vi "OpenDrive.vi"(8 "error in":errorcluster) -> (0 "error out":errorcluster, 2 "Calibrated":bool, 3 "RobotDriveDevRef":T1={"DevStatus"={"status"=FALSE, "code"=0, "source"=""}, "Motors[]"=[], "Square Inputs"=FALSE, "Max Output"=1.0})   [LabVIEW 2020]
uses:
  <vilib>/Rock Robotics/WPI/RobotDrive/WPI_RobotDriveDevRef.ctl
  <vilib>/Rock Robotics/WPI/MotorControl/WPI_MotorControlDeviceRef.ctl
  <vilib>/Rock Robotics/WPI/MotorControl/WPI_MotorControlType.ctl
  <vilib>/Rock Robotics/SystemInterfaces/DIO/FPGA_DIOPWMChannel.ctl
  <vilib>/Rock Robotics/WPI/PWM/WPI_PWMDeadband.ctl
  <vilib>/Rock Robotics/SystemInterfaces/DIO/FPGA_DIOChannel.ctl
  <vilib>/Rock Robotics/WPI/ThirdParty/Phoenix-LabVIEW/Motor Controller/Controls/CTRE_Phoenix_MotorControl_NeutralMode.ctl
  <vilib>/Rock Robotics/WPI/Encoder/WPI_EncoderType.ctl
  <vilib>/Rock Robotics/WPI/SafetyOutput/WPI_SafetyOutputConfigMenu.ctl
  <vilib>/Rock Robotics/WPI/Counter/WPI_CounterDigitalInputToDigitalSource.vi
  <vilib>/Rock Robotics/WPI/Counter/WPI_CounterOpen Semi Period Mode.vi
  <vilib>/Rock Robotics/WPI/RobotDrive/WPI_RobotDriveOpen2MotorWithExistingMotors.vi
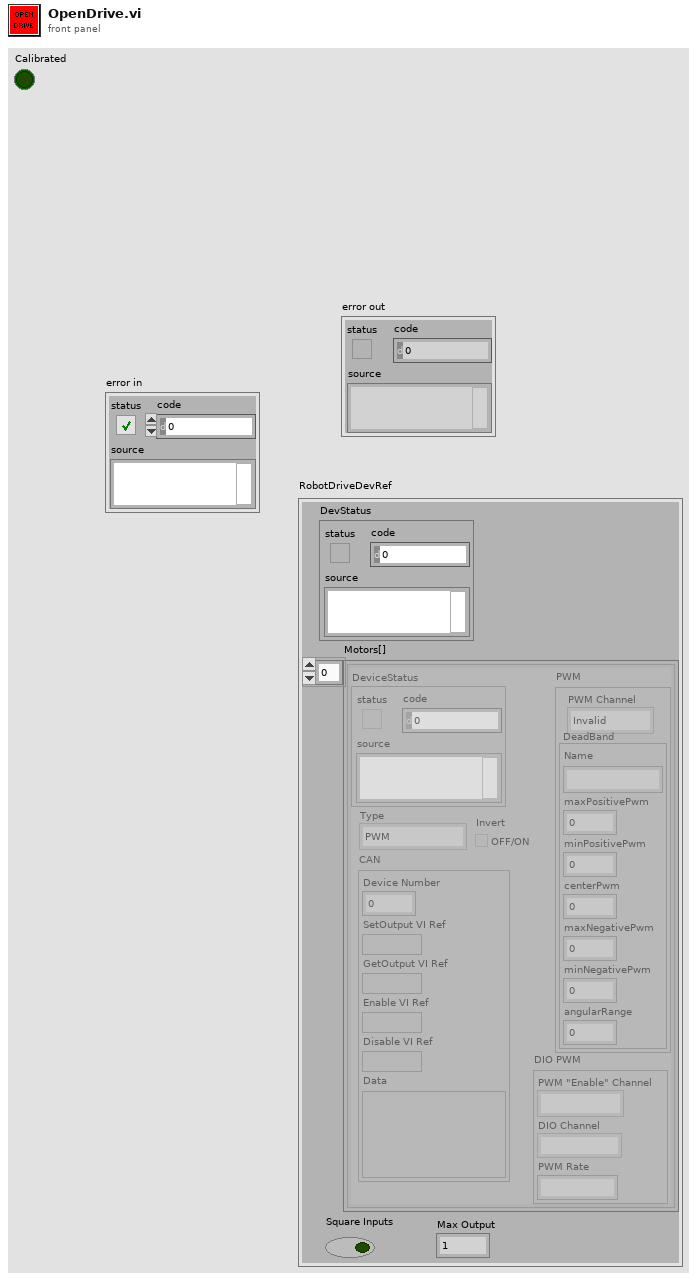
[diagram p1: front panel]
types:
  T1 = typedef "WPI_RobotDriveDevRef.ctl" = cluster{"DevStatus":errorcluster, "Motors[]":T2[], "Square Inputs":bool, "Max Output":dbl}
  T2 = typedef "WPI_MotorControlDeviceRef.ctl" = cluster{"DeviceStatus":errorcluster, "Type":T3, "PWM":cluster{"PWM Channel":T4, "DeadBand":T5}, "CAN":cluster{"Device Number":u8, "SetOutput VI Ref":variant, "GetOutput VI Ref":variant, "Enable VI Ref":variant, "Disable VI Ref":variant, "Data":variant}, "Invert":bool, "DIO PWM":cluster{"PWM \"Enable\" Channel":T4, "DIOChannel":T6, "PWM Rate":dbl}}
  T3 = typedef "WPI_MotorControlType.ctl" = enum16{"PWM", "CAN", "DIO PWM"}
  T4 = typedef "FPGA_DIOPWMChannel.ctl" = enum8{"PWM 0", "PWM 1", "PWM 2", "PWM 3", "PWM 4", "PWM 5", "PWM 6", "PWM 7", "PWM 8", "PWM 9", "PWM MXP 0", "PWM MXP 1", "PWM MXP 2", "PWM MXP 3", "PWM MXP 4", "PWM MXP 5", "PWM MXP 6", "PWM MXP 7", "PWM MXP 8", "PWM MXP 9", "Invalid"}
  T5 = typedef "WPI_PWMDeadband.ctl" = cluster{"Name":string, "maxPositivePwm":i32, "minPositivePwm":i32, "centerPwm":i32, "maxNegativePwm":i32, "minNegativePwm":i32, "angularRange":u16}
  T6 = typedef "FPGA_DIOChannel.ctl" = enum8{"DIO 0", "DIO 1", "DIO 2", "DIO 3", "DIO 4", "DIO 5", "DIO 6", "DIO 7", "DIO 8", "DIO 9", "DIO MXP 0", "DIO MXP 1", "DIO MXP 2", "DIO MXP 3", "DIO MXP 4", "DIO MXP 5", "DIO MXP 6", "DIO MXP 7", "DIO MXP 8", "DIO MXP 9", "DIO MXP 10", "DIO MXP 11", "DIO MXP 12", "DIO MXP 13", "DIO MXP 14", "DIO MXP 15", "SPI Port CS1", "SPI Port CS2", "SPI Port CS3", "SPI Port MISO", "SPI Port MOSI", "Invalid"}
  T7 = typedef "CTRE_Phoenix_MotorControl_NeutralMode.ctl" = enum8{"EEPROMSetting", "Override to Coast", "Override to Brake"}
  T8 = typedef "WPI_EncoderType.ctl" = enum16{"1x", "2x", "4x"}
  T9 = typedef "WPI_SafetyOutputConfigMenu.ctl" = enum16{"Enable", "Disable"}
  T10 = typedef "WPI_DigitalInputDevRef.ctl" = cluster{"DevStatus":errorcluster, "DIO Channel":T6}
  T11 = typedef "FPGA_CounterEncoderSourceConvertionLVSourceType.ctl" = cluster{"DevStatus":errorcluster, "AnalogTriggerMode?":bool, "DigitalMode":cluster{"DIO Channel":T12}, "AnalogTriggerMode":cluster{"AnalogTriggerIndex":T13, "OutputType":T14}}
  T12 = typedef "FPGA_DIODigitalSourceChannel.ctl" = enum8{"DIO 0", "DIO 1", "DIO 2", "DIO 3", "DIO 4", "DIO 5", "DIO 6", "DIO 7", "DIO 8", "DIO 9", "DIO MXP 0", "DIO MXP 1", "DIO MXP 2", "DIO MXP 3", "DIO MXP 4", "DIO MXP 5", "DIO MXP 6", "DIO MXP 7", "DIO MXP 8", "DIO MXP 9", "DIO MXP 10", "DIO MXP 11", "DIO MXP 12", "DIO MXP 13", "DIO MXP 14", "DIO MXP 15", "SPI Port CS1", "SPI Port CS2", "SPI Port CS3", "SPI Port MISO", "SPI Port MOSI", "Disabled"}
  T13 = typedef "FPGA_AnalogTriggerIndex.ctl" = enum8{"Trig 0", "Trig 1", "Trig 2", "Trig 3", "Trig 4", "Trig 5", "Trig 6", "Trig 7", "Invalid"}
  T14 = typedef "FPGA_AnalogTriggerOutType.ctl" = enum16{"InWindow", "TriggerState", "Rising", "Falling"}
  T15 = typedef "WPI_CounterDevRef.ctl" = cluster{"DevStatus":errorcluster, "CntIndex":T16}
  T16 = typedef "FPGA_CounterCtrSystemIndex.ctl" = enum8{"Ctr 0", "Ctr 1", "Ctr 2", "Ctr 3", "Ctr 4", "Ctr 5", "Ctr 6", "Ctr 7", "Invalid"}
  T17 = typedef "WPI_EncoderDevRef.ctl" = cluster{"DevStatus":errorcluster, "EncoderIndex":T18, "CounterIndex":T16, "DistancePerCount":dbl, "Decoding Type":T8}
  T18 = typedef "FPGA_EncoderIdx.ctl" = enum8{"Enc 0", "Enc 1", "Enc 2", "Enc 3", "Enc 4", "Enc 5", "Enc 6", "Enc 7", "Invalid"}
  T19 = typedef "ADIS16470 Device Reference.ctl" = cluster{"DevStatus":errorcluster, "Hardware Config":T20, "Calibration Complete":refnum<notifier>, "Status Reference":refnum<data-value>, "Data Reference":refnum<data-value>, "Sychronous Process VI":T23, "Cmd FIFO":refnum<k33>, "Source":T11, "Data FIFO":refnum<k33>, "Calibration Time (ms)":u32, "Data Reference":refnum<data-value>}
  T20 = typedef "ADIS16470 Hardware Configuration.ctl" = cluster{"SPI Clock Rate (Hz)":dbl, "IMU SPI Mode (3)":T21, "IMU Reset Pin":T6, "IMU SPI Bus":T22, "IMU Data Ready Pin":T6, "Stall Config":cluster{"Pow2BytesPerRead":u8, "StallTicks":u16, "CsToSclkTicks":u8}}
  T21 = typedef "WPI_SPIMode.ctl" = enum16{"Mode 0 (Clk Idle Low,Sample on Leading)", "Mode 1 (Clk Idle Low,Sample on Trailing)", "Mode 2 (Clk Idle High,Sample on Leading)", "Mode 3 (Clk Idle High,Sample on Trailing)"}
  T22 = typedef "spi_bus.ctl" = enum16{"SPI On-Board, CS0", "SPI On-Board, CS1", "SPI On-Board, CS2", "SPI On-Board, CS3", "SPI MXP", "Invalid"}
  T23 = typedef "ADIS16470 Process.ctl" = refnum<vi>
  T24 = typedef "ADIS16470 Status.ctl" = cluster{"Calibrated?":bool, "IMU Detected?":bool}
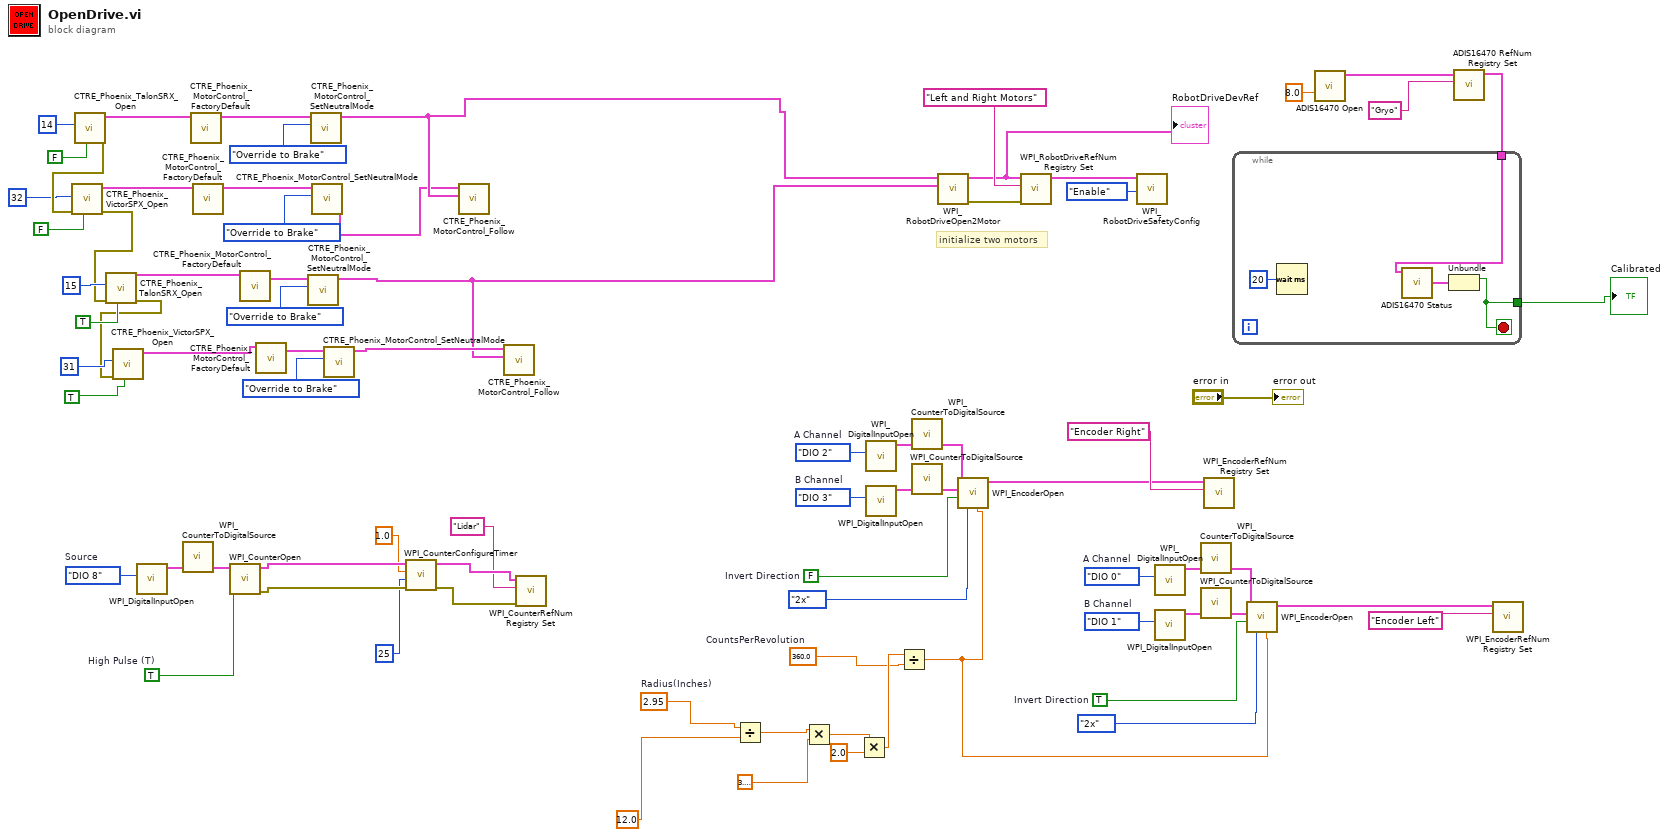
[diagram p0: block diagram]
diagram:
  w29 = TRUE  # High Pulse (T)
  w38 = FPGA_DIOChannel."DIO 8"  # Source
  w43 = 2.95  # Radius(Inches)
  w53 = TRUE  # Invert Direction
  w57 = FPGA_DIOChannel."DIO 1"  # B Channel
  w56 = FPGA_DIOChannel."DIO 0"  # A Channel
  w45 = 360.0  # CountsPerRevolution
  w63 = FALSE  # Invert Direction
  w67 = FPGA_DIOChannel."DIO 3"  # B Channel
  w66 = FPGA_DIOChannel."DIO 2"  # A Channel
  # "initialize two motors"
  n1 = call <vilib>:"CTRE_Phoenix_TalonSRX_Open.vi"("Invert"=FALSE, "Device Number"=u8 14) -> ("error out"=w15:errorcluster, "PhoenixMotorControlDevRef"=w20:T2)  [unwired: 8 in]
  n2 = call <vilib>:"CTRE_Phoenix_VictorSPX_Open.vi"("Invert"=FALSE, "error in"=w15, "Device Number"=u8 32) -> ("error out"=w14:errorcluster, "PhoenixMotorControlDevRef"=w11:T2)  [unwired: 7 in]
  n3 = call <vilib>:"CTRE_Phoenix_TalonSRX_Open.vi"("Invert"=TRUE, "error in"=w14, "Device Number"=u8 15) -> ("error out"=w7:errorcluster, "PhoenixMotorControlDevRef"=w26:T2)  [unwired: 7 in]
  n4 = call <vilib>:"CTRE_Phoenix_VictorSPX_Open.vi"("Invert"=TRUE, "error in"=w7, "Device Number"=u8 31) -> ("PhoenixMotorControlDevRef"=w10:T2)  [unwired: 7 in, 1 out]
  n5 = call <vilib>:"WPI_DigitalInputOpen.vi"("DIO Channel"=w38) -> ("DigitalInputDevRef"=w37:T10)  [unwired: 1 in, 9 out]
  n6 = call-poly <vilib>:"WPI_CounterToDigitalSource.vi"("DigitalInputDevRef"=w37) -> ("Digital Source"=w39:T11)  [unwired: 6 out]
  n7 = call <vilib>:"CTRE_Phoenix_MotorControl_FactoryDefault.vi"("PhoenixMotorControlDevRef"=w20) -> ("PhoenixMotorControlDevRef"=w21:T2)  [unwired: 9 in, 1 out]
  n8 = call <vilib>:"CTRE_Phoenix_MotorControl_FactoryDefault.vi"("PhoenixMotorControlDevRef"=w11) -> ("PhoenixMotorControlDevRef"=w17:T2)  [unwired: 9 in, 1 out]
  n9 = call-poly <vilib>:"WPI_CounterOpen.vi"("High Pulse (T)"=w29, "Source"=w39) -> ("error out"=w33:errorcluster, "CounterDevRef"=w36:T15)  [unwired: 3 in, 5 out]
  n10 = call <vilib>:"CTRE_Phoenix_MotorControl_FactoryDefault.vi"("PhoenixMotorControlDevRef"=w26) -> ("PhoenixMotorControlDevRef"=w27:T2)  [unwired: 9 in, 1 out]
  n11 = call <vilib>:"CTRE_Phoenix_MotorControl_FactoryDefault.vi"("PhoenixMotorControlDevRef"=w10) -> ("PhoenixMotorControlDevRef"=w24:T2)  [unwired: 9 in, 1 out]
  n12 = call <vilib>:"CTRE_Phoenix_MotorControl_SetNeutralMode.vi"("Motor Control Neutral Mode"=CTRE_Phoenix_MotorControl_NeutralMode."Override to Brake", "PhoenixMotorControlDevRef"=w27) -> ("PhoenixMotorControlDevRef"=w6:T2)  [unwired: 8 in, 1 out]
  n13 = call <vilib>:"CTRE_Phoenix_MotorControl_SetNeutralMode.vi"("Motor Control Neutral Mode"=CTRE_Phoenix_MotorControl_NeutralMode."Override to Brake", "PhoenixMotorControlDevRef"=w21) -> ("PhoenixMotorControlDevRef"=w19:T2)  [unwired: 8 in, 1 out]
  n14 = call <vilib>:"CTRE_Phoenix_MotorControl_SetNeutralMode.vi"("Motor Control Neutral Mode"=CTRE_Phoenix_MotorControl_NeutralMode."Override to Brake", "PhoenixMotorControlDevRef"=w17) -> ("PhoenixMotorControlDevRef"=w16:T2)  [unwired: 8 in, 1 out]
  n15 = call <vilib>:"CTRE_Phoenix_MotorControl_SetNeutralMode.vi"("Motor Control Neutral Mode"=CTRE_Phoenix_MotorControl_NeutralMode."Override to Brake", "PhoenixMotorControlDevRef"=w24) -> ("PhoenixMotorControlDevRef"=w23:T2)  [unwired: 8 in, 1 out]
  n16 = call <vilib>:"WPI_CounterConfigureTimer.vi"("error in (no error)"=w33, "Number Samples to Average"=u8 25, "MaxPeriod (sec)"=1.0, "CounterDevRef in"=w36) -> ("error out"=w32:errorcluster, "CounterDevRef out"=w35:T15)  [unwired: 6 in]
  n17 = call <vilib>:"CTRE_Phoenix_MotorControl_Follow.vi"("Master Controller to Follow"=w19, "PhoenixMotorControlDevRef"=w16) -> ()  [unwired: 8 in, 2 out]
  n18 = call <vilib>:"CTRE_Phoenix_MotorControl_Follow.vi"("Master Controller to Follow"=w6, "PhoenixMotorControlDevRef"=w23) -> ()  [unwired: 8 in, 2 out]
  n19 = call <vilib>:"WPI_CounterRefNum Registry Set.vi"("error in (no error)"=w32, "refnum name"="Lidar", "CounterDevRef"=w35) -> ()  [unwired: 7 in, 2 out]
  n20 = Divide(x=w43, y=12.0) -> (x/y=w42:dbl)
  n21 = Multiply(x=w42, y=3.141592653589793) -> (x*y=w48:dbl)
  n22 = Multiply(x=w48, y=2.0) -> (x*y=w46:dbl)
  n23 = call <vilib>:"WPI_DigitalInputOpen.vi"("DIO Channel"=w66) -> ("DigitalInputDevRef"=w64:T10)  [unwired: 1 in, 9 out]
  n24 = call <vilib>:"WPI_DigitalInputOpen.vi"("DIO Channel"=w67) -> ("DigitalInputDevRef"=w65:T10)  [unwired: 1 in, 9 out]
  n25 = Divide(x=w46, y=w45) -> (x/y=w41:dbl)
  n26 = call-poly <vilib>:"WPI_CounterToDigitalSource.vi"("DigitalInputDevRef"=w64) -> ("Digital Source"=w68:T11)  [unwired: 6 out]
  n27 = call-poly <vilib>:"WPI_CounterToDigitalSource.vi"("DigitalInputDevRef"=w65) -> ("Digital Source"=w69:T11)  [unwired: 6 out]
  n28 = call-poly <vilib>:"WPI_RobotDriveOpen2Motor.vi"("Right Motor Dev Ref"=w6, "Left Motor Dev Ref"=w19) -> ("error out"=w72:errorcluster, "RobotDriveDevRef"=w70:T1)  [unwired: 3 in, 5 out]
  "RobotDriveDevRef" <- w70
  n29 = call <vilib>:"WPI_EncoderOpen.vi"("DistancePerCount"=w41, "Decoding Type"=WPI_EncoderType."2x", "Invert Direction (False)"=w63, "BSource"=w69, "ASource"=w68) -> ("EncoderDevRef"=w60:T17)  [unwired: 5 in, 1 out]
  n30 = call <vilib>:"WPI_RobotDriveRefNum Registry Set.vi"("error in (no error)"=w72, "refnum name"="Left and Right Motors", "RobotDriveDevRef"=w70) -> ("RobotDriveDevRef"=w73:T1)  [unwired: 1 in, 7 out]
  n31 = call <vilib>:"WPI_RobotDriveSafetyConfig.vi"("mode"=WPI_SafetyOutputConfigMenu."Enable", "RobotDriveDevRef"=w73) -> ()  [unwired: 8 in, 2 out]
  n32 = call <vilib>:"WPI_DigitalInputOpen.vi"("DIO Channel"=w56) -> ("DigitalInputDevRef"=w54:T10)  [unwired: 1 in, 9 out]
  n33 = call <vilib>:"WPI_DigitalInputOpen.vi"("DIO Channel"=w57) -> ("DigitalInputDevRef"=w55:T10)  [unwired: 1 in, 9 out]
  n34 = call-poly <vilib>:"WPI_CounterToDigitalSource.vi"("DigitalInputDevRef"=w54) -> ("Digital Source"=w58:T11)  [unwired: 6 out]
  n35 = call-poly <vilib>:"WPI_CounterToDigitalSource.vi"("DigitalInputDevRef"=w55) -> ("Digital Source"=w59:T11)  [unwired: 6 out]
  n36 = call <vilib>:"WPI_EncoderRefNum Registry Set.vi"("refnum name"="Encoder Right", "EncoderDevRef"=w60) -> ()  [unwired: 8 in, 2 out]
  n37 = call <vilib>:"WPI_EncoderOpen.vi"("DistancePerCount"=w41, "Decoding Type"=WPI_EncoderType."2x", "Invert Direction (False)"=w53, "BSource"=w59, "ASource"=w58) -> ("EncoderDevRef"=w50:T17)  [unwired: 5 in, 1 out]
  n38 = call <vilib>:"ADIS16470 Open.vi"("Initial Calibration Time (4s)"=8.0) -> ("ADIS16470DevRef"=w4:T19)  [unwired: 9 in, 1 out]
  n39 = call <vilib>:"ADIS16470 RefNum Registry Set.vi"("refnum name"="Gryo", "ADIS16470DevRef in"=w4) -> ("ADIS16470DevRef out"=w1:T19)  [unwired: 8 in, 1 out]
  n40 = while {
    tunnel: [w81] -> w5
    tunnel: w1 -> [w80]
    stop <- w81 stop-if-true
    n41 = Wait (ms)(milliseconds to wait=u32 20) -> ()  [unwired: 1 out]
    n42 = call <vilib>:"ADIS16470 Status.vi"("ADIS16470DevRef"=w80) -> ("ADIS16470 Status"=w82:T24)  [unwired: 8 in, 2 out]
    n43 = Unbundle(w82) -> ("Calibrated?"=w81:bool)  [unwired: 1 out]
  }
  "Calibrated" <- w5
  n44 = call <vilib>:"WPI_EncoderRefNum Registry Set.vi"("refnum name"="Encoder Left", "EncoderDevRef"=w50) -> ()  [unwired: 8 in, 2 out]
  "error out" <- "error in"
